vi "Error站_ResetFlag.vi"(0 "ref in":T1, 2 "FlagArray":bool[](array[boolean]), 3 "error in":errorcluster) -> (6 "ref out":T1, 9 "error out":errorcluster)   [LabVIEW 2015]
panel:
  out "Timed out":bool
  in  "ms timeout (-1)":i32=-1
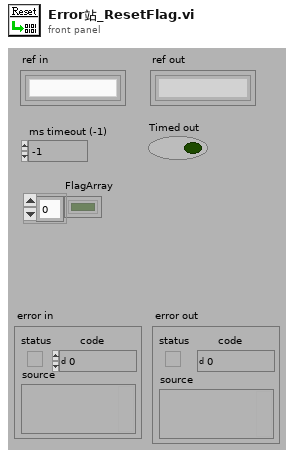
[diagram p1: front panel]
types:
  T1 = typedef "Error站_ref.ctl" = refnum<k1>
  T2 = typedef "Error站_Flag.ctl" = cluster{"0":bool, "1":bool, "2":bool, "3":bool, "4":bool, "5":bool, "6":bool, "7":bool, "8":bool, "9":bool, "10":bool, "11":bool, "12":bool, "13":bool, "14":bool, "15":bool, "16":bool, "17":bool, "18":bool, "19":bool, "20":bool, "21":bool, "22":bool, "23":bool, "24":bool, "25":bool, "26":bool, "27":bool, "28":bool, "29":bool}
  T3 = enum16{"OpenReference", "CloseReference", "Get Data", "Set Data", "Set Flag"}
  T4 = typedef "Semaphore RefNum" = refnum<k1>
  T5 = cluster{"FlagArray[0]":bool, "FlagArray[1]":bool, "FlagArray[2]":bool, "FlagArray[3]":bool, "FlagArray[4]":bool, "FlagArray[5]":bool, "FlagArray[6]":bool, "FlagArray[7]":bool, "FlagArray[8]":bool, "FlagArray[9]":bool, "FlagArray[10]":bool, "FlagArray[11]":bool, "FlagArray[12]":bool, "FlagArray[13]":bool, "FlagArray[14]":bool, "FlagArray[15]":bool, "FlagArray[16]":bool, "FlagArray[17]":bool, "FlagArray[18]":bool, "FlagArray[19]":bool, "FlagArray[20]":bool, "FlagArray[21]":bool, "FlagArray[22]":bool, "FlagArray[23]":bool, "FlagArray[24]":bool, "FlagArray[25]":bool, "FlagArray[26]":bool, "FlagArray[27]":bool, "FlagArray[28]":bool, "FlagArray[29]":bool}
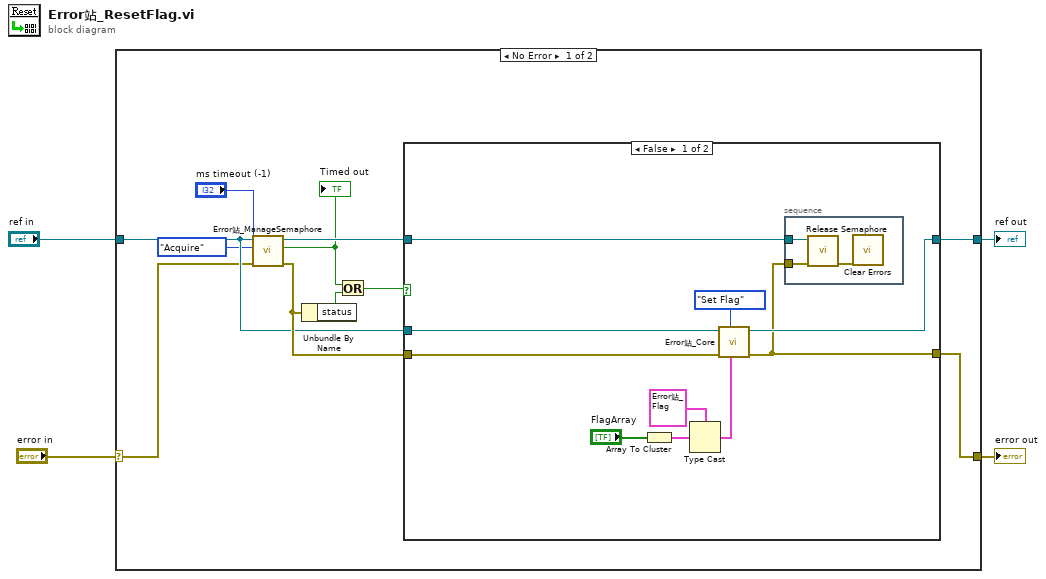
[diagram p0: block diagram]
diagram:
  n1 = case shown="No Error" "error in" {
    selector: "error in" -> [w6 w32]
    tunnel: [w10 w32] -> w3
    tunnel: "ref in" -> [w11 w31]
    tunnel: [w12 w31] -> w1
    frame No Error {
      n2 = call "Error站_ManageSemaphore.vi"("error in (no error)"=w6, "ms timeout (-1)"="ms timeout (-1)", "Method (Acquire)"=enum8{"Acquire", "Destroy"}."Acquire", "ref"=w11) -> ("error out"=w15:errorcluster, "Timed out"=w7:bool, "semaphore out"=w13:T4)  [unwired: 1 in]
      "Timed out" <- w7
      n3 = Unbundle By Name(w15) -> ("status"=w8:bool)
      n4 = Or(x=w7, y=w8) -> (x .or. y?=w14:bool)
      n5 = case shown="False" w14 {
        tunnel: [w24 w29] -> w12
        tunnel: w13 -> [w25 _]
        tunnel: w15 -> [w22 w30]
        tunnel: [w23 w30] -> w10
        tunnel: w11 -> [w20 w29]
        frame False {
          n6 = Array To Cluster(array="FlagArray") -> (cluster=w18:T5)
          n7 = Type Cast(type=T2 {"0"=FALSE, "1"=FALSE, "2"=FALSE, "3"=FALSE, "4"=FALSE, "5"=FALSE, "6"=FALSE, "7"=FALSE, "8"=FALSE, "9"=FALSE, "10"=FALSE, "11"=FALSE, "12"=FALSE, "13"=FALSE, "14"=FALSE, "15"=FALSE, "16"=FALSE, "17"=FALSE, "18"=FALSE, "19"=FALSE, "20"=FALSE, "21"=FALSE, "22"=FALSE, "23"=FALSE, "24"=FALSE, "25"=FALSE, "26"=FALSE, "27"=FALSE, "28"=FALSE, "29"=FALSE} ("LoadTray_Flag"), x=w18) -> (*(type *) &x=w17:T2)
          n8 = call "Error站_Core.vi"("Flag in"=w17, "Function"=T3."Set Flag", "error in"=w22, "ref in"=w20) -> ("error out"=w23:errorcluster, "ref out"=w24:T1)  [unwired: 4 in, 2 out]
          n9 = stacked-sequence {
            tunnel: w25 -> [w28]
            tunnel: w23 -> [w26]
            frame #0 {
              n10 = call <vilib>:"Release Semaphore.vi"("error in (no error)"=w26, "semaphore"=w28) -> ("error out"=w27:errorcluster)  [unwired: 4 in, 1 out]
              n11 = call <vilib>:"Clear Errors.vi"("error in (no error)"=w27) -> ()  [unwired: 5 in, 2 out]
            }
          }
        }
        frame True {
        }
      }
    }
    frame Error {
    }
  }
  "error out" <- w3
  "ref out" <- w1
